vi "Write ES Data to Optimization.vi"(7 "Bus by ID":T1[](array[typedef]), 8 "error in":errorcluster, 11 "Generic Optimization in":refnum<class "Generic Optimization.lvclass">) -> (0 "error out":errorcluster, 3 "Generic Optimization out":refnum<class "Generic Optimization.lvclass">)   [LabVIEW 2018, in "Generic Optimization Actor.lvlib" / "Generic Optimization.lvclass"]
uses:
  Generic Optimization.lvclass
  C:/Users/Administrator/Desktop/2018LabVIEW EMS/EMS Generic Actor/EMS Generic/EMS Generic.lvclass
  Optimization Controls/Bus by ID.ctl
  <vilib>/ORNL/CSEISMIC DDS/CSEISMIC DDS Base/Data Types/Controls/DeviceID.ctl
  EMS Generic Actor/EMS Generic/EMS Generic.lvclass/EMS Generic.ctl
  <vilib>/ORNL/CSEISMIC DDS/CSEISMIC DDS Base/Data Types/ES_Info.ctl
  <vilib>/ORNL/CSEISMIC DDS/CSEISMIC DDS Base/Data Types/Controls/EfficiencyCurve.ctl
  <vilib>/ORNL/CSEISMIC DDS/CSEISMIC DDS Base/Data Types/ES_Measurement.ctl
  <vilib>/ORNL/CSEISMIC DDS/CSEISMIC DDS Base/Data Types/DER_Info.ctl
  EMS Generic Actor/EMS Generic/EMS Generic.lvclass
  <vilib>/ORNL/CSEISMIC DDS/CSEISMIC DDS Base/CSEISMIC DDS.lvclass
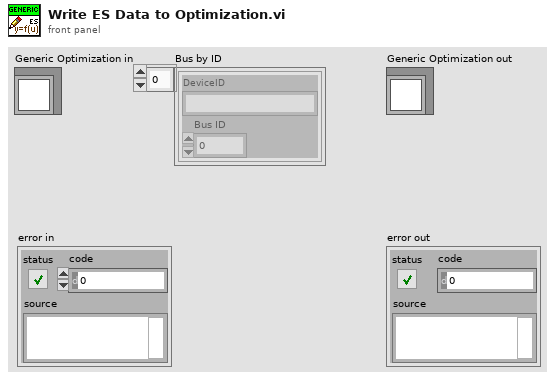
[diagram p1: front panel]
types:
  T1 = typedef "Generic Optimization Actor.lvlib/Generic Optimization.lvclass/Bus by ID.ctl" = cluster{"DeviceID":T2, "Bus ID":dbl}
  T2 = typedef "CSEISMIC DDS.lvlib/CSEISMIC DDS.lvclass/DeviceID.ctl" = string
  T3 = typedef "CSEISMIC DDS.lvlib/CSEISMIC DDS.lvclass/DER_Info.ctl" = cluster{"DeviceID":T2, "LineConfig":u8[], "NominalVoltage(V)":dbl, "PowerRating(kVA)":dbl, "VFControl":bool, "PControl":bool, "QControl":bool, "PFControl":bool, "PVControl":bool, "Droop":bool, "DroopConfigurable":bool, "Unbalanced":bool}
  T4 = typedef "CSEISMIC DDS.lvlib/CSEISMIC DDS.lvclass/ES_Measurement.ctl" = cluster{"DeviceID":T2, "SOC (%)":dbl}
  T5 = typedef "CSEISMIC DDS.lvlib/CSEISMIC DDS.lvclass/ES_Info.ctl" = cluster{"DeviceID":T2, "EnergyRating (kWh)":dbl, "RampRate (kW/s)":dbl, "MaxPowerFactorLeading":dbl, "MaxPowerFactorLagging":dbl, "ChargingEfficiencyCurve":T6, "DischargingEfficiencyCurve":T6, "MinSOC (%)":dbl, "MaxSOC (%)":dbl}
  T6 = typedef "CSEISMIC DDS.lvlib/CSEISMIC DDS.lvclass/EfficiencyCurve.ctl" = cluster{"Power (kW)":dbl[], "Efficiency (%)":dbl[]}
  T7 = typedef "EMS Generic Actor.lvlib/EMS Generic.lvclass/Data Type DVRs.ctl" = cluster{"IED_Status":refnum<data-value>, "IED_Status_0":refnum<data-value>, "DER_Measurement":refnum<data-value>, "DER_Info":refnum<data-value>, "DER_Status":refnum<data-value>, "ES_Measurement":refnum<data-value>, "ES_Info":refnum<data-value>, "PV_Info":refnum<data-value>, "SmartRelay_Info":refnum<data-value>, "SmartRelay_Measurement":refnum<data-value>, "Meter_Info":refnum<data-value>, "Meter_Measurement":refnum<data-value>, "HVAC_Status":refnum<data-value>, "HVAC_Measurement":refnum<data-value>, "PriceData_RealTime":refnum<data-value>, "PriceData_Demand":refnum<data-value>, "PriceData_Energy":refnum<data-value>, "ForecastData_Long":refnum<data-value>, "ForecastData_Short":refnum<data-value>, "DER_Control":refnum<data-value>, "DER_SetPointF":refnum<data-value>, "DER_SetPointP":refnum<data-value>, "DER_SetPointQ":refnum<data-value>, "DER_SetPointPF":refnum<data-value>, "DER_SetPointV":refnum<data-value>, "PV_setCurtailment":refnum<data-value>, "PV_setRampRate":refnum<data-value>, "Relay_Control":refnum<data-value>, "Load_Control":refnum<data-value>, "HVAC_Control":refnum<data-value>, "Generator_Info":refnum<data-value>, "ForecastData_Long_Backup":refnum<data-value>, "PriceData_RealTime_Backup":refnum<data-value>}
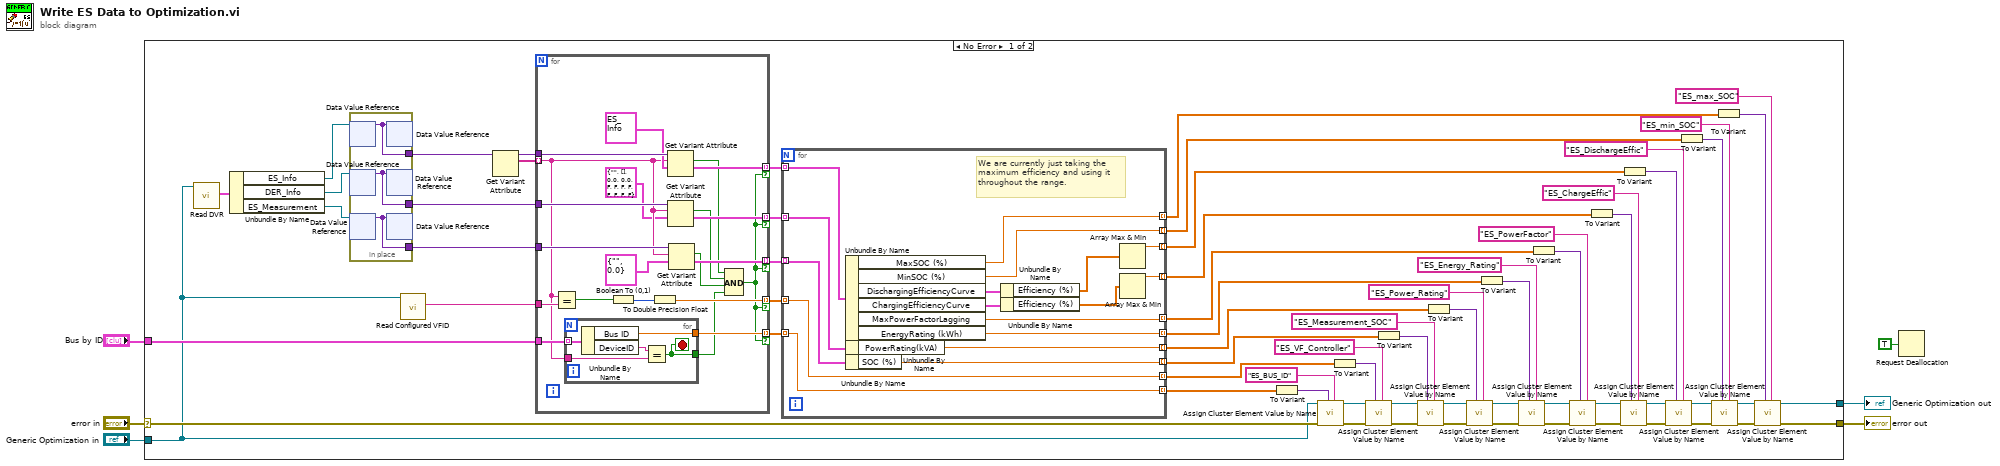
[diagram p0: block diagram]
diagram:
  n1 = case shown="No Error" "error in" {
    selector: "error in" -> [w47 w122]
    tunnel: [w68 w122] -> w6
    tunnel: [w8 w121] -> w4
    tunnel: "Generic Optimization in" -> [w7 w121]
    tunnel: "Bus by ID" -> [w13 _]
    frame No Error {
      n2 = call "Read DVR.vi"("EMS Generic in"=w7) -> ("DVR"=w24:T7)  [unwired: 9 in, 1 out]
      n3 = Unbundle By Name(w24) -> ("ES_Info"=w23:refnum<data-value>, "DER_Info"=w12:refnum<data-value>, "ES_Measurement"=w21:refnum<data-value>)
      n4 = in-place {
        in-place-border: [w120] -> w22
        in-place-border: [w119] -> w19
        in-place-border: [w118] -> w11
        n5 = in-place-dvr #1(w23) -> (w120:variant)  [unwired: 1 out]
        n6 = in-place-dvr #2(w12) -> (w118:variant)  [unwired: 1 out]
        n7 = in-place-dvr #3(w21) -> (w119:variant)  [unwired: 1 out]
        n8 = in-place-dvr #1(w120) -> ()  [unwired: 2 out]
        n9 = in-place-dvr #2(w118) -> ()  [unwired: 2 out]
        n10 = in-place-dvr #3(w119) -> ()  [unwired: 2 out]
      }
      n11 = call "Read Configured VFID.vi"("EMS Generic in"=w7) -> ("VFID"=w9:T2)  [unwired: 8 in, 2 out]
      n12 = Get Variant Attribute(Variant=w22) -> (duplicate Variant=w20:variant, names=w18:string[])  [unwired: 3 in, 2 out]
      n13 = for {
        tunnel: w18 -> [w99] mode=indexing
        tunnel: w20 -> [w112]
        tunnel: w9 -> [w110]
        tunnel: w13 -> [w108]
        tunnel: w19 -> [w107]
        tunnel: [w104] -> w15 mode=indexing if=w92
        tunnel: [w103] -> w16 mode=indexing if=w92
        tunnel: [w102] -> w17 mode=indexing if=w92
        tunnel: [w101] -> w14 mode=indexing if=w92
        tunnel: w11 -> [w100]
        tunnel: [w97] -> w10 mode=indexing if=w92
        n14 = Equal?(x=w99, y=w110) -> (x = y?=w105:bool)
        n15 = for {
          tunnel: w108 -> [w117] mode=indexing
          tunnel: w99 -> [w116]
          tunnel: [w114] -> w101
          tunnel: [w113] -> w96
          stop <- w113 stop-if-true
          n16 = Unbundle By Name(w117) -> ("Bus ID"=w114:dbl, "DeviceID"=w115:T2)
          n17 = Equal?(x=w115, y=w116) -> (x = y?=w113:bool)
        }
        n18 = Boolean To (0,1)(Boolean=w105) -> (0, 1=w106:i16)
        n19 = To Double Precision Float(number=w106) -> (double precision float=w104:dbl)
        n20 = Get Variant Attribute(Variant=w112, name=w99, default value (empty Variant)=T5 {"DeviceID"="", "EnergyRating (kWh)"=0.0, "RampRate (kW/s)"=0.0, "MaxPowerFactorLeading"=0.0, "MaxPowerFactorLagging"=0.0, "ChargingEfficiencyCurve"={"Power (kW)"=[], "Efficiency (%)"=[]}, "DischargingEfficiencyCurve"={"Power (kW)"=[], "Efficiency (%)"=[]}, "MinSOC (%)"=0.0, "MaxSOC (%)"=0.0} ("ES_Info")) -> (found=w95:bool, value=w102:T5)  [unwired: 1 in, 2 out]
        n21 = Get Variant Attribute(Variant=w100, name=w99, default value (empty Variant)=T3 {"DeviceID"="", "LineConfig"=[], "NominalVoltage(V)"=0.0, "PowerRating(kVA)"=0.0, "VFControl"=FALSE, "PControl"=FALSE, "QControl"=FALSE, "PFControl"=FALSE, "PVControl"=FALSE, "Droop"=FALSE, "DroopConfigurable"=FALSE, "Unbalanced"=FALSE} ("DER_Info")) -> (found=w94:bool, value=w97:T3)  [unwired: 1 in, 2 out]
        n22 = Get Variant Attribute(Variant=w107, name=w99, default value (empty Variant)=T4 {"DeviceID"="", "SOC (%)"=0.0} ("ES_Measurement")) -> (found=w93:bool, value=w103:T4)  [unwired: 1 in, 2 out]
        n23 = Compound Arithmetic op=AND(w95, w94, w93, w96) -> (w92:bool)
      }
      n24 = for {
        tunnel: [w81] -> w34 mode=indexing
        tunnel: [w80] -> w33 mode=indexing
        tunnel: [w78] -> w32 mode=indexing
        tunnel: [w75] -> w31 mode=indexing
        tunnel: [w91] -> w30 mode=indexing
        tunnel: [w90] -> w29 mode=indexing
        tunnel: [w88] -> w28 mode=indexing
        tunnel: [w87] -> w27 mode=indexing
        tunnel: [w85] -> w26 mode=indexing
        tunnel: [w82] -> w25 mode=indexing
        tunnel: w17 -> [w77] mode=indexing
        tunnel: w16 -> [w79] mode=indexing
        tunnel: w15 -> [w80] mode=indexing
        tunnel: w14 -> [w81] mode=indexing
        tunnel: w10 -> [w76] mode=indexing
        # "We are currently just taking the maximum efficiency and using it throughout the range."
        n25 = Unbundle By Name(w77) -> ("MaxSOC (%)"=w87:dbl, "MinSOC (%)"=w88:dbl, "DischargingEfficiencyCurve"=w89:T6, "ChargingEfficiencyCurve"=w84:T6, "MaxPowerFactorLagging"=w90:dbl, "EnergyRating (kWh)"=w91:dbl)
        n26 = Unbundle By Name(w76) -> ("PowerRating(kVA)"=w75:dbl)
        n27 = Unbundle By Name(w79) -> ("SOC (%)"=w78:dbl)
        n28 = Unbundle By Name(w89) -> ("Efficiency (%)"=w86:dbl[])
        n29 = Unbundle By Name(w84) -> ("Efficiency (%)"=w83:dbl[])
        n30 = Array Max & Min(array=w86) -> (max value=w85:dbl)  [unwired: 3 out]
        n31 = Array Max & Min(array=w83) -> (max value=w82:dbl)  [unwired: 3 out]
      }
      n32 = To Variant(anything=w34) -> (Variant=w35:variant)
      n33 = call "Assign Cluster Element Value by Name.vi"("Element Name"="ES_BUS_ID" ("Keyword Name"), "Value"=w35, "error in"=w47, "Generic Optimization"=w7) -> ("error out"=w71:errorcluster, "Generic Optimization out"=w73:refnum<class "Generic Optimization.lvclass">)  [unwired: 6 in]
      n34 = To Variant(anything=w33) -> (Variant=w69:variant)
      n35 = call "Assign Cluster Element Value by Name.vi"("Element Name"="ES_VF_Controller" ("Keyword Name"), "Value"=w69, "error in"=w71, "Generic Optimization"=w73) -> ("error out"=w72:errorcluster, "Generic Optimization out"=w74:refnum<class "Generic Optimization.lvclass">)  [unwired: 6 in]
      n36 = To Variant(anything=w32) -> (Variant=w37:variant)
      n37 = call "Assign Cluster Element Value by Name.vi"("Element Name"="ES_Measurement_SOC" ("Keyword Name"), "Value"=w37, "error in"=w72, "Generic Optimization"=w74) -> ("error out"=w46:errorcluster, "Generic Optimization out"=w43:refnum<class "Generic Optimization.lvclass">)  [unwired: 6 in]
      n38 = To Variant(anything=w31) -> (Variant=w39:variant)
      n39 = call "Assign Cluster Element Value by Name.vi"("Element Name"="ES_Power_Rating" ("Keyword Name"), "Value"=w39, "error in"=w46, "Generic Optimization"=w43) -> ("error out"=w45:errorcluster, "Generic Optimization out"=w44:refnum<class "Generic Optimization.lvclass">)  [unwired: 6 in]
      n40 = To Variant(anything=w30) -> (Variant=w41:variant)
      n41 = call "Assign Cluster Element Value by Name.vi"("Element Name"="ES_Energy_Rating" ("Keyword Name"), "Value"=w41, "error in"=w45, "Generic Optimization"=w44) -> ("error out"=w57:errorcluster, "Generic Optimization out"=w56:refnum<class "Generic Optimization.lvclass">)  [unwired: 6 in]
      n42 = To Variant(anything=w29) -> (Variant=w48:variant)
      n43 = call "Assign Cluster Element Value by Name.vi"("Element Name"="ES_PowerFactor" ("Keyword Name"), "Value"=w48, "error in"=w57, "Generic Optimization"=w56) -> ("error out"=w61:errorcluster, "Generic Optimization out"=w60:refnum<class "Generic Optimization.lvclass">)  [unwired: 6 in]
      n44 = To Variant(anything=w25) -> (Variant=w50:variant)
      n45 = call "Assign Cluster Element Value by Name.vi"("Element Name"="ES_ChargeEffic" ("Keyword Name"), "Value"=w50, "error in"=w61, "Generic Optimization"=w60) -> ("error out"=w62:errorcluster, "Generic Optimization out"=w59:refnum<class "Generic Optimization.lvclass">)  [unwired: 6 in]
      n46 = To Variant(anything=w26) -> (Variant=w52:variant)
      n47 = call "Assign Cluster Element Value by Name.vi"("Element Name"="ES_DischargeEffic" ("Keyword Name"), "Value"=w52, "error in"=w62, "Generic Optimization"=w59) -> ("error out"=w63:errorcluster, "Generic Optimization out"=w58:refnum<class "Generic Optimization.lvclass">)  [unwired: 6 in]
      n48 = To Variant(anything=w28) -> (Variant=w54:variant)
      n49 = call "Assign Cluster Element Value by Name.vi"("Element Name"="ES_min_SOC" ("Keyword Name"), "Value"=w54, "error in"=w63, "Generic Optimization"=w58) -> ("error out"=w67:errorcluster, "Generic Optimization out"=w66:refnum<class "Generic Optimization.lvclass">)  [unwired: 6 in]
      n50 = To Variant(anything=w27) -> (Variant=w64:variant)
      n51 = call "Assign Cluster Element Value by Name.vi"("Element Name"="ES_max_SOC" ("Keyword Name"), "Value"=w64, "error in"=w67, "Generic Optimization"=w66) -> ("error out"=w68:errorcluster, "Generic Optimization out"=w8:refnum<class "Generic Optimization.lvclass">)  [unwired: 6 in]
    }
    frame Error {
    }
  }
  "error out" <- w6
  "Generic Optimization out" <- w4
  n52 = Request Deallocation(TRUE ("flag")) -> ()
